vi "QuerySystemDefinitionFile.vi"(8 "error in (no error)":errorcluster, 11 "System Definiton File in":path) -> (0 "error out":errorcluster, 3 "System Definition Information out":T1)   [LabVIEW 2015, in "VeriStandTestUtilities.lvlib"]
uses:
  VeriStandTestUtilities.lvlib
  SystemDefinitionInformation.ctl
  TargetInformation.ctl
  ChassisInformation.ctl
  NationalInstruments.VeriStand.SystemDefinitionAPI
  <userlib>/_OpenG.lib/file/file.llb/Append Path to Root if Relative - Scalar__ogtk.vi
panel:
  in  "System Definition Information":T1
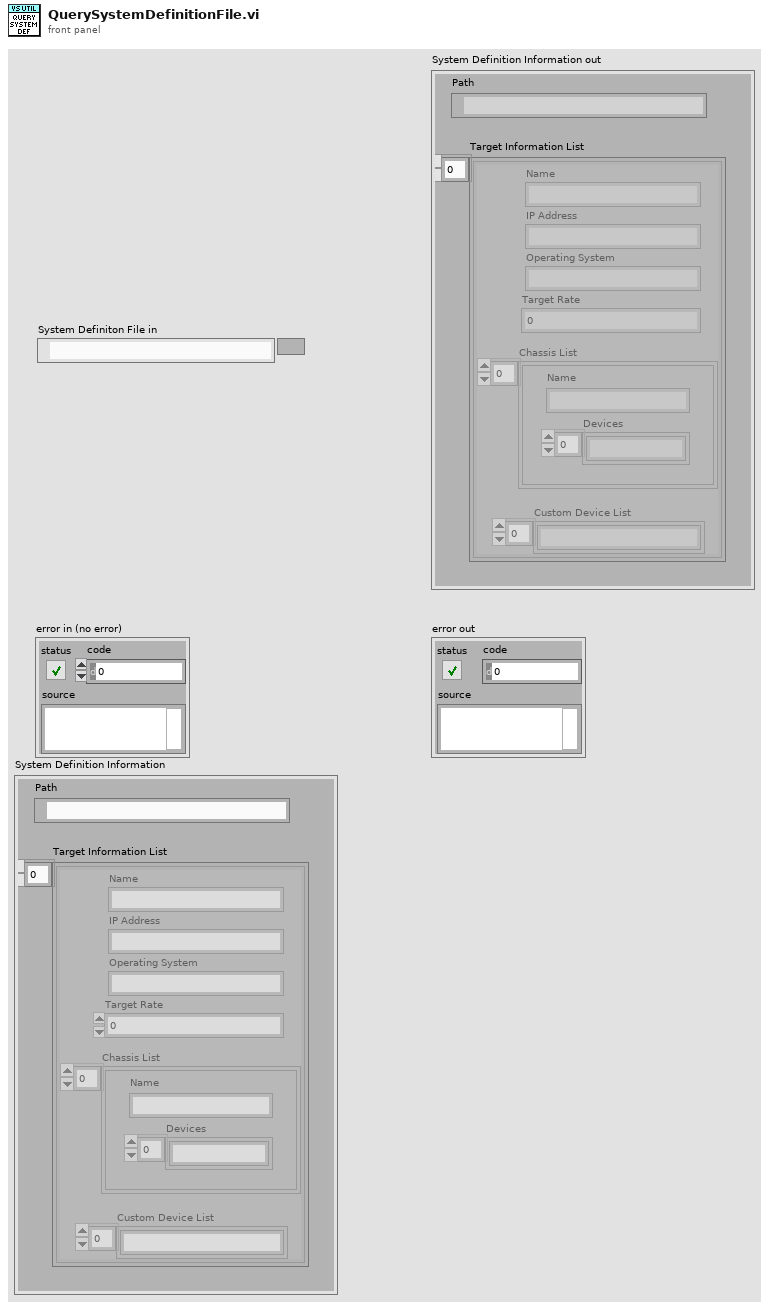
[diagram p1: front panel]
types:
  T1 = typedef "VeriStandTestUtilities.lvlib/SystemDefinitionInformation.ctl" = cluster{"Path":path, "Target Information List":T2[]}
  T2 = typedef "VeriStandTestUtilities.lvlib/TargetInformation.ctl" = cluster{"Name":string, "IP Address":string, "Operating System":string, "Target Rate":dbl, "Chassis List":T3[], "Custom Device List":string[]}
  T3 = typedef "VeriStandTestUtilities.lvlib/ChassisInformation.ctl" = cluster{"Name":string, "Devices":string[]}
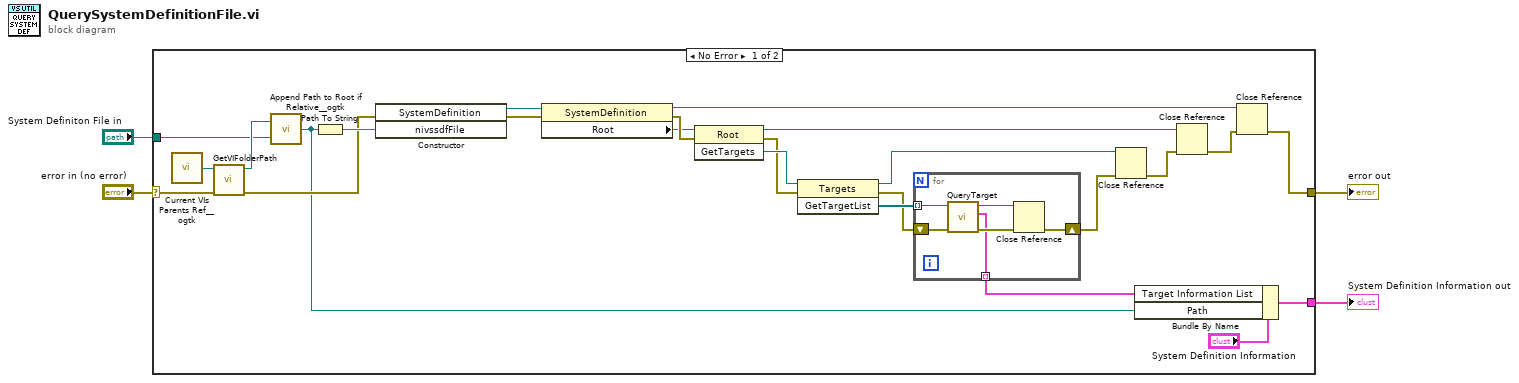
[diagram p0: block diagram]
diagram:
  n1 = case shown="No Error" "error in (no error)" {
    selector: "error in (no error)" -> [w12 w36]
    tunnel: [w17 w36] -> w3
    tunnel: "System Definiton File in" -> [w9 _]
    tunnel: [w5 _] -> w1
    frame No Error {
      n2 = call <userlib>:"Current VIs Parents Ref__ogtk.vi"() -> ("Calling VI's Reference"=w13:refnum<vi>)  [unwired: 2 in]
      n3 = call "GetVIFolderPath.vi"("error in (no error)"=w12, "VI Reference in"=w13) -> ("error out"=w11:errorcluster, "VI Folder Path out"=w10:path)  [unwired: 8 in]
      n4 = call-poly <userlib>:"Append Path to Root if Relative__ogtk.vi"("Absolute or Relative Path"=w9, "Root Path"=w10) -> ("Absolute or Appended Path"=w7:path)
      n5 = Path To String(path=w7) -> (string=w18:string)
      n6 = constructor class="SystemDefinition"(error in=w11, "nivssdfFile"=w18) -> (reference out=w26:refnum<k24>, error out=w25:errorcluster)  [unwired: 2 in, 2 out]
      n7 = property class="SystemDefinition"(reference=w26, error in=w25) -> (reference out=w20:refnum<k24>, error out=w28:errorcluster, "Root"=w27:refnum<k24>)
      n8 = invoke class="Root" method="GetTargets"(reference=w27, error in=w28) -> (reference out=w21:refnum<k24>, error out=w24:errorcluster, "GetTargets"=w29:refnum<k24>)  [unwired: 1 in]
      n9 = invoke class="Targets" method="GetTargetList"(reference=w29, error in=w24) -> (reference out=w23:refnum<k24>, error out=w15:errorcluster, "GetTargetList"=w16:refnum<k24>[])  [unwired: 1 in]
      n10 = for {
        tunnel: w16 -> [w32] mode=indexing
        shift-right: [w33] -> w14
        shift-left: w15 -> [w35]
        tunnel: [w30] -> w6 mode=indexing
        n11 = call "QueryTarget.vi"("error in (no error)"=w35, "Target Reference in"=w32) -> ("error out"=w34:errorcluster, "Target Information"=w30:T2, "Target Reference out"=w31:refnum<k24>)  [unwired: 7 in]
        n12 = Close Reference(reference=w31, error in (no error)=w34) -> (error out=w33:errorcluster)
      }
      n13 = Close Reference(reference=w23, error in (no error)=w14) -> (error out=w22:errorcluster)
      n14 = Bundle By Name(cluster="System Definition Information", "Target Information List"=w6, "Path"=w7) -> (w5:T1)
      n15 = Close Reference(reference=w21, error in (no error)=w22) -> (error out=w19:errorcluster)
      n16 = Close Reference(reference=w20, error in (no error)=w19) -> (error out=w17:errorcluster)
    }
    frame Error {
    }
  }
  "error out" <- w3
  "System Definition Information out" <- w1
